vi "tanh.vi"(1 "x":dbl[][](array[numeric])) -> (0 "y":T1)   [LabVIEW 2020]
uses:
  <vilib>/Analysis/Matrix/Datatypes/RealMatrix.ctl
  <vilib>/Analysis/Matrix/Numeric/Conversions/Array To Matrix - RA.vi
  <vilib>/Analysis/Matrix/NI_Matrix.lvlib
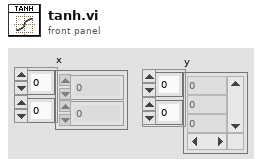
[diagram p1: front panel]
types:
  T1 = typedef "NI_Matrix.lvlib/RealMatrix.ctl" = dbl[][]
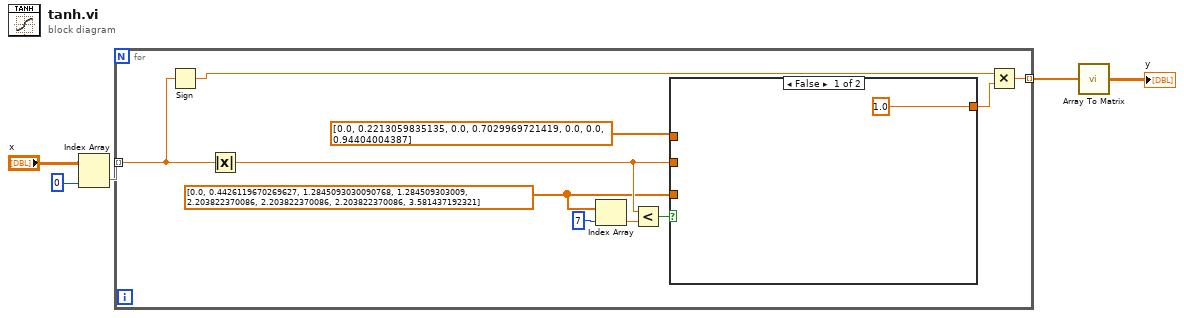
[diagram p0: block diagram]
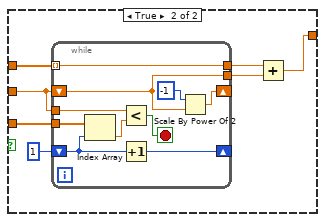
[diagram p2: hidden frame]
diagram:
  n1 = Index Array(array="x", index (col)=0) -> (element=w3:dbl[])  [unwired: 1 in]
  n2 = for {
    tunnel: w3 -> [w11] mode=indexing
    tunnel: [w8] -> w2 mode=indexing
    w7 = dbl[] [0.0, 0.4426119670269627, 1.2845093030090768, 1.284509303009, 2.203822370086, 2.203822370086, 2.203822370086, 3.581437192321]
    n3 = Sign(1:w11) -> (0:w10:dbl)
    n4 = Absolute Value(x=w11) -> (abs(x)=w12:dbl)
    n5 = Index Array(array=w7, index=7) -> (element=w14:dbl)
    n6 = Less?(x=w12, y=w14) -> (x < y?=w15:bool)
    n7 = case shown="False" w15 {
      tunnel: w12 -> [_ w22]
      tunnel: [1.0 w21] -> w9
      tunnel: w7 -> [_ w20]
      tunnel: dbl[] [0.0, 0.2213059835135, 0.0, 0.7029969721419, 0.0, 0.0, 0.94404004387] -> [_ w19]
      frame False {
      }
      frame True {
        n8 = while {
          tunnel: w22 -> [w33]
          shift-right: [w31] -> _
          shift-left: 1 -> [w29]
          shift-right: [w28] -> _
          shift-left: w22 -> [w26]
          tunnel: [w26] -> w18
          tunnel: w20 -> [w25]
          tunnel: [w24] -> w17
          tunnel: w19 -> [w24] mode=indexing
          stop <- w32 stop-if-true
          n9 = Index Array(array=w25, index=w29) -> (element=w30:dbl)
          n10 = Less?(x=w33, y=w30) -> (x < y?=w32:bool)
          n11 = Increment(x=w29) -> (x+1=w31:i32)
          n12 = Scale By Power Of 2(n=-1, x=w26) -> (x*2^n=w28:dbl)
        }
        n13 = Add(x=w17, y=w18) -> (x+y=w21:dbl)
      }
    }
    n14 = Multiply(x=w10, y=w9) -> (x*y=w8:dbl)
  }
  n15 = call-poly <vilib>:"Array To Matrix.vi"("Real 1D Array"=w2) -> ("Real Matrix (Column Vector)"=→"y":T1)
